vi "Create ALL Documentation.vi"(0 "Target Folder":path, 1 "Library Palette Icon":path, 2 "Library Examples Folder":path, 3 "Library Description":string, 5 "VI Paths":T1(array[cluster]), 7 "Supplimental VI Information":string="Use the dictionary reference when calling other <a href=\"Dictionary.html\">Dictionary</a> functions.", 9 "Library Name":string, 11 "error in (no error)":errorcluster, 12 "Template VI HTML Doc":path, 13 "Template Library HTML Doc":path, 14 "Library Documentation":string) -> (15 "error out":errorcluster)   [LabVIEW 2011]
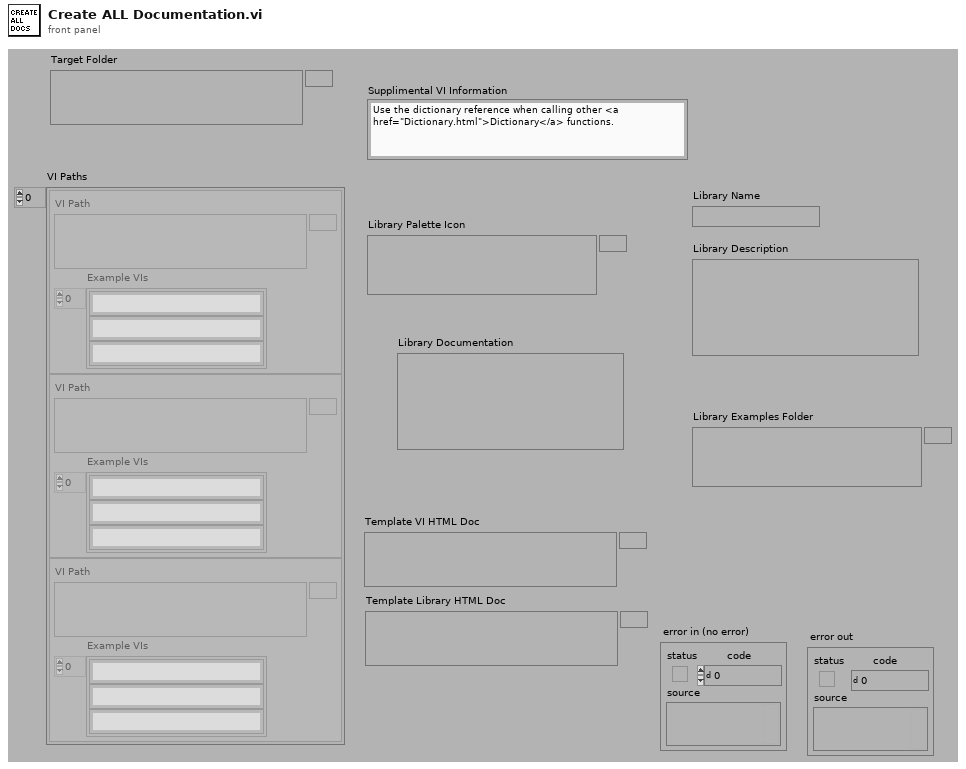
[diagram p1: front panel]
types:
  T1 = cluster{"VI Path":path, "Example VIs":string[]}[]
  T2 = cluster{"Function Rows":string, "Library Name":string, "VI Doc Path":string, "Library Examples Folder":string, "Library Examples Folder Escaped":string, "Library Description":string, "Library Palette Image Path":string, "Library Documentation":string}
  T3 = cluster{"VI Name":string, "VI Description":string, "VI Doc Path":string}
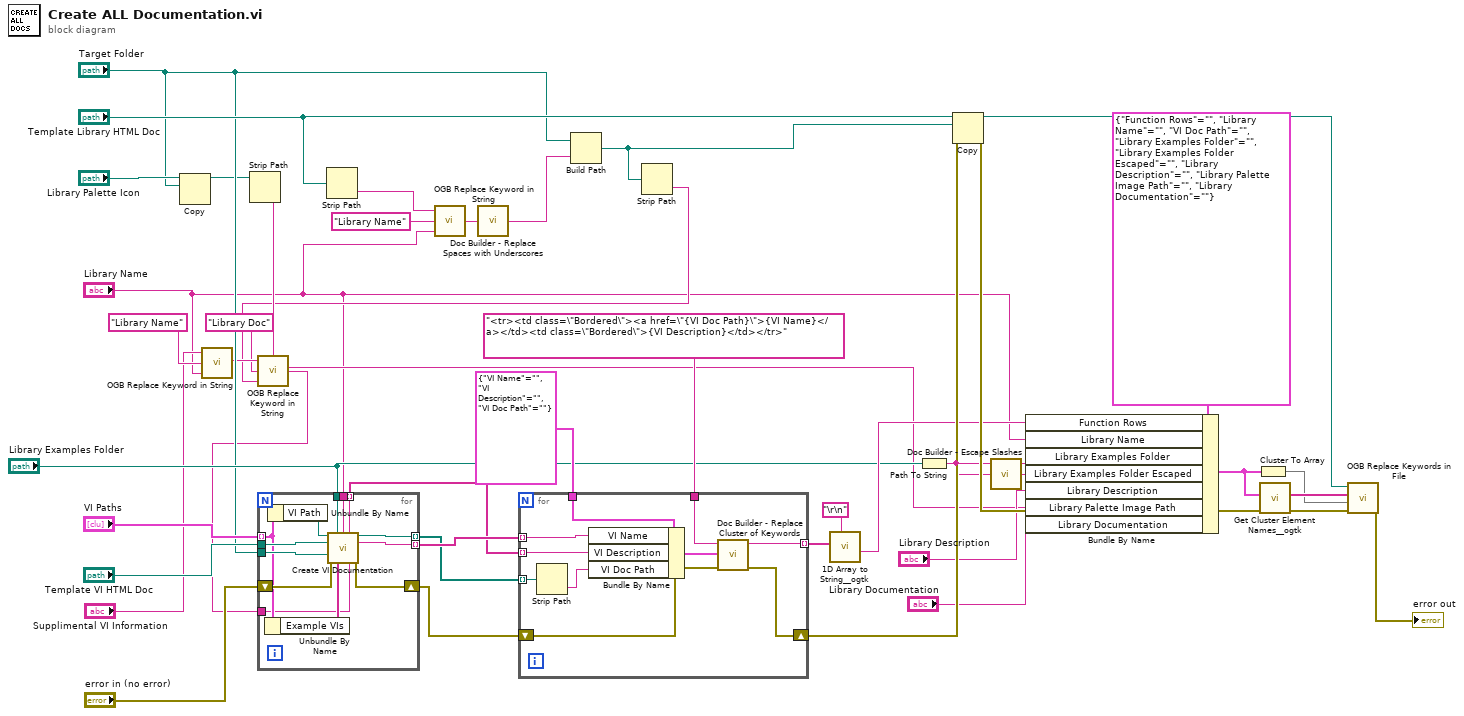
[diagram p0: block diagram]
diagram:
  n1 = Copy(10:"Target Folder", 11:"Library Palette Icon") -> (3:w11:path)  [unwired: 3 in, 2 out]
  n2 = call "OGB Replace Keyword in String.vi"("Value"="Library Name", "Keyword"="Library Name", "String"="Supplimental VI Information") -> ("String out"=w8:string)
  n3 = Strip Path(path=w11) -> (name=w10:string)  [unwired: 1 out]
  n4 = Strip Path(path="Template Library HTML Doc") -> (name=w32:string)  [unwired: 1 out]
  n5 = call "OGB Replace Keyword in String.vi"("Value"="Library Name", "Keyword"="Library Name", "String"=w32) -> ("String out"=w18:string)
  n6 = call "Doc Builder - Replace Spaces with Underscores.vi"("String"=w18) -> ("String out"=w3:string)  [unwired: 4 in]
  n7 = Build Path(base path="Target Folder", name or relative path=w3) -> (appended path=w30:path)
  n8 = Strip Path(path=w30) -> (name=w6:string)  [unwired: 1 out]
  n9 = call "OGB Replace Keyword in String.vi"("Value"=w6, "Keyword"="Library Doc", "String"=w8) -> ("String out"=w4:string)
  n10 = for {
    tunnel: "VI Paths" -> [w47] mode=indexing
    tunnel: "Template VI HTML Doc" -> [w56]
    tunnel: "Target Folder" -> [w55]
    tunnel: [w54] -> w36 mode=indexing
    tunnel: [w53] -> w38 mode=indexing
    shift-right: [w52] -> w33
    shift-left: "error in (no error)" -> [w51]
    tunnel: [w50] -> w37 mode=indexing
    tunnel: "Library Examples Folder" -> [w49]
    tunnel: w4 -> [w45]
    tunnel: "Library Name" -> [w44]
    n11 = Unbundle By Name(w47) -> ("Example VIs"=w46:string[])
    n12 = Unbundle By Name(w47) -> ("VI Path"=w48:path)
    n13 = call "Create VI Documentation.vi"("VI Path"=w48, "Library Examples Folder"=w49, "Library Name"=w44, "Template VI HTML Doc"=w56, "Target Folder"=w55, "error in (no error)"=w51, "Example VIs"=w46, "Supplimental VI Information"=w45) -> ("VI Description"=w50:string, "HTML file path"=w54:path, "VI Name"=w53:string, "error out"=w52:errorcluster)  [unwired: 4 in]
  }
  n14 = for {
    tunnel: "<tr><td class=\"Bordered\"><a href=\"{VI Doc Path}\">{VI Name}</a></td><td class=\"Bordered\">{VI Description}</td></tr>" -> [w61]
    tunnel: T3 {"VI Name"="", "VI Description"="", "VI Doc Path"=""} -> [w66]
    tunnel: w38 -> [w65] mode=indexing
    tunnel: w37 -> [w64] mode=indexing
    tunnel: w36 -> [w63] mode=indexing
    tunnel: [w60] -> w35 mode=indexing
    shift-right: [w59] -> w29
    shift-left: w33 -> [w58]
    n15 = Strip Path(path=w63) -> (name=w62:string)  [unwired: 1 out]
    n16 = Bundle By Name(cluster=w66, "VI Name"=w65, "VI Description"=w64, "VI Doc Path"=w62) -> (w57:T3)
    n17 = call "Doc Builder - Replace Cluster of Keywords.vi"("error in (no error)"=w58, "VCluster of KeyVals"=w57, "String"=w61) -> ("error out"=w59:errorcluster, "String out"=w60:string)  [unwired: 7 in]
  }
  n18 = call <userlib>:"1D Array to String__ogtk.vi"("delimiter (Tab)"="\r\n", "Array of Strings"=w35) -> ("delimited string"=w21:string)  [unwired: 9 in]
  n19 = Path To String(path="Library Examples Folder") -> (string=w17:string)
  n20 = Copy(8:w29, 10:w30, 11:"Template Library HTML Doc") -> (0:w24:errorcluster, 3:w28:path)  [unwired: 2 in, 1 out]
  n21 = call "Doc Builder - Escape Slashes.vi"("String"=w17) -> ("String out"=w16:string)  [unwired: 4 in]
  n22 = Bundle By Name(cluster=T2 {"Function Rows"="", "Library Name"="", "VI Doc Path"="", "Library Examples Folder"="", "Library Examples Folder Escaped"="", "Library Description"="", "Library Palette Image Path"="", "Library Documentation"=""}, "Function Rows"=w21, "Library Name"="Library Name", "Library Examples Folder"=w17, "Library Examples Folder Escaped"=w16, "Library Description"="Library Description", "Library Palette Image Path"=w10, "Library Documentation"="Library Documentation") -> (w20:T2)
  n23 = Cluster To Array(cluster=w20) -> (array=w26:string[])
  n24 = call <userlib>:"Get Cluster Element Names__ogtk.vi"("error in (no error)"=w24, "Cluster"=w20) -> ("error out"=w25:errorcluster, "Element Names"=w27:string[])  [unwired: 8 in]
  n25 = call "OGB Replace Keywords in File.vi"("error in (no error)"=w25, "Values"=w26, "Keywords"=w27, "file path"=w28) -> ("error out"=→"error out":errorcluster)  [unwired: 6 in, 1 out]
